vi "웨더.vi"() -> ()   [LabVIEW 2014]
panel:
  out "문자열":string
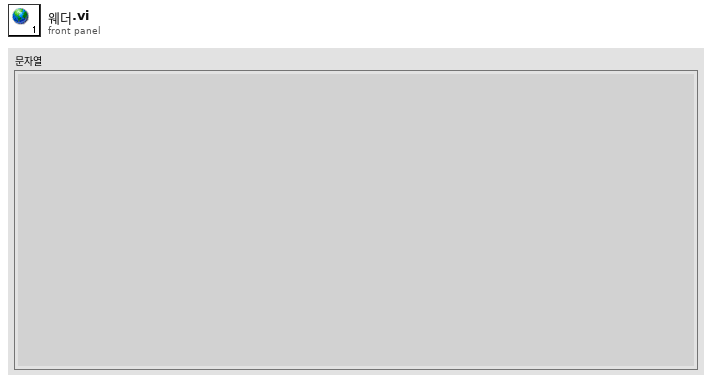
[diagram p1: front panel]
diagram:
